vi "FPGAQueuesTest.vi"   [LabVIEW 2014]
uses:
  <vilib>/rvi/LocalResourceManager/LocalResourceManager.xnode
  <vilib>/rvi/DataTransferAndStorage/Container/Common/niFpgaContainerGetUniqueNameForEmu.vi
  <vilib>/rvi/DataTransferAndStorage/Container/Common/niFpgaContainerSetEmuInfo.vi
  <vilib>/rvi/eio/common/nirviEmuReportErrorAndStop.vi
  <vilib>/rvi/DataTransferAndStorage/Container/XNode/niFpgaContainer.xnode
  <vilib>/rvi/FIFO/Fifo_Resource/niFpgaFifoEmulationRefIn.vi
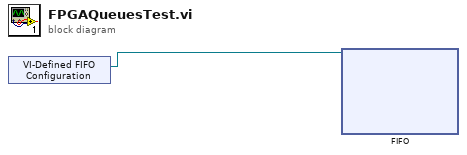
[diagram p0: block diagram]
diagram:
  n1 = xnode "VI-Defined FIFO Configuration"() -> ("FIFO Out"=w1:refnum<k21>)
  n2 = xnode "FIFO"("FIFO In"=w1) -> ()  [unwired: 2 in, 2 out]
